vi "LVDatasetTest.vi"() -> ()   [LabVIEW 2011]
uses:
  JelmersTracker.llb/TrackerDLL.vi
  <vilib>/Utility/file.llb/Read From Spreadsheet File (DBL).vi
  <vilib>/Utility/file.llb/Write To Spreadsheet File (DBL).vi
panel:
  out "C++ QI error":cluster{dbl, dbl}(graph)
  out "LV Z":cluster{"Normalized Z":sgl, sgl}(graph)
  out "True pos":dbl(graph)
  out "LV ZLUT":dbl[][](graph)
  out "JTrk ZLUT":sgl[][](graph)
  in  "XCorWindow":u32=64
  out "FPS":dbl
  in  "Use LV tracker":bool=TRUE
  in  "xcor profile":i32=32
  in  "result output dir":string="dataset_result\\roi80"
  out "LV COM error":cluster{dbl, dbl}(graph)
  out "LV QI error":cluster{dbl, dbl}(graph)
  out "LV XCor X&Y error":cluster{dbl, dbl}(graph)
  out "X Resolution":i32
  out "Image Type":T1 items=["Grayscale (U8)", "Grayscale (I16)", "Grayscale (SGL)", "Complex (CSG)", "RGB (U32)", "HSL (U32)", "RGB (U64)", "Grayscale (U16)"]
  in  "LVTracker settings":T2={"Rmax (pix)"=50, "RminZ (pix)"=5, "angular pixel\n coverage factor"=0.7, "radial pixel\n coverage factor"=3.0}
  out "Debug output":sgl[][](graph)
  out "COM X & Y error":cluster{dbl, dbl}(graph)
  out "text file path":path
  out "File":string caption="Result"
  in  "Image count":i32=200
  out "Image":T3(plugin-control)
  in  "xcor_iterations":i32=1
  out "Radial profile":sgl[](graph)
  in  "Path":path=path "D:/jcnossen1/ztracker/Qpaper_007LUT_varyRoi80/tmp_002"
  in  "Browse?":bool=TRUE
  in  "debug library":bool=TRUE
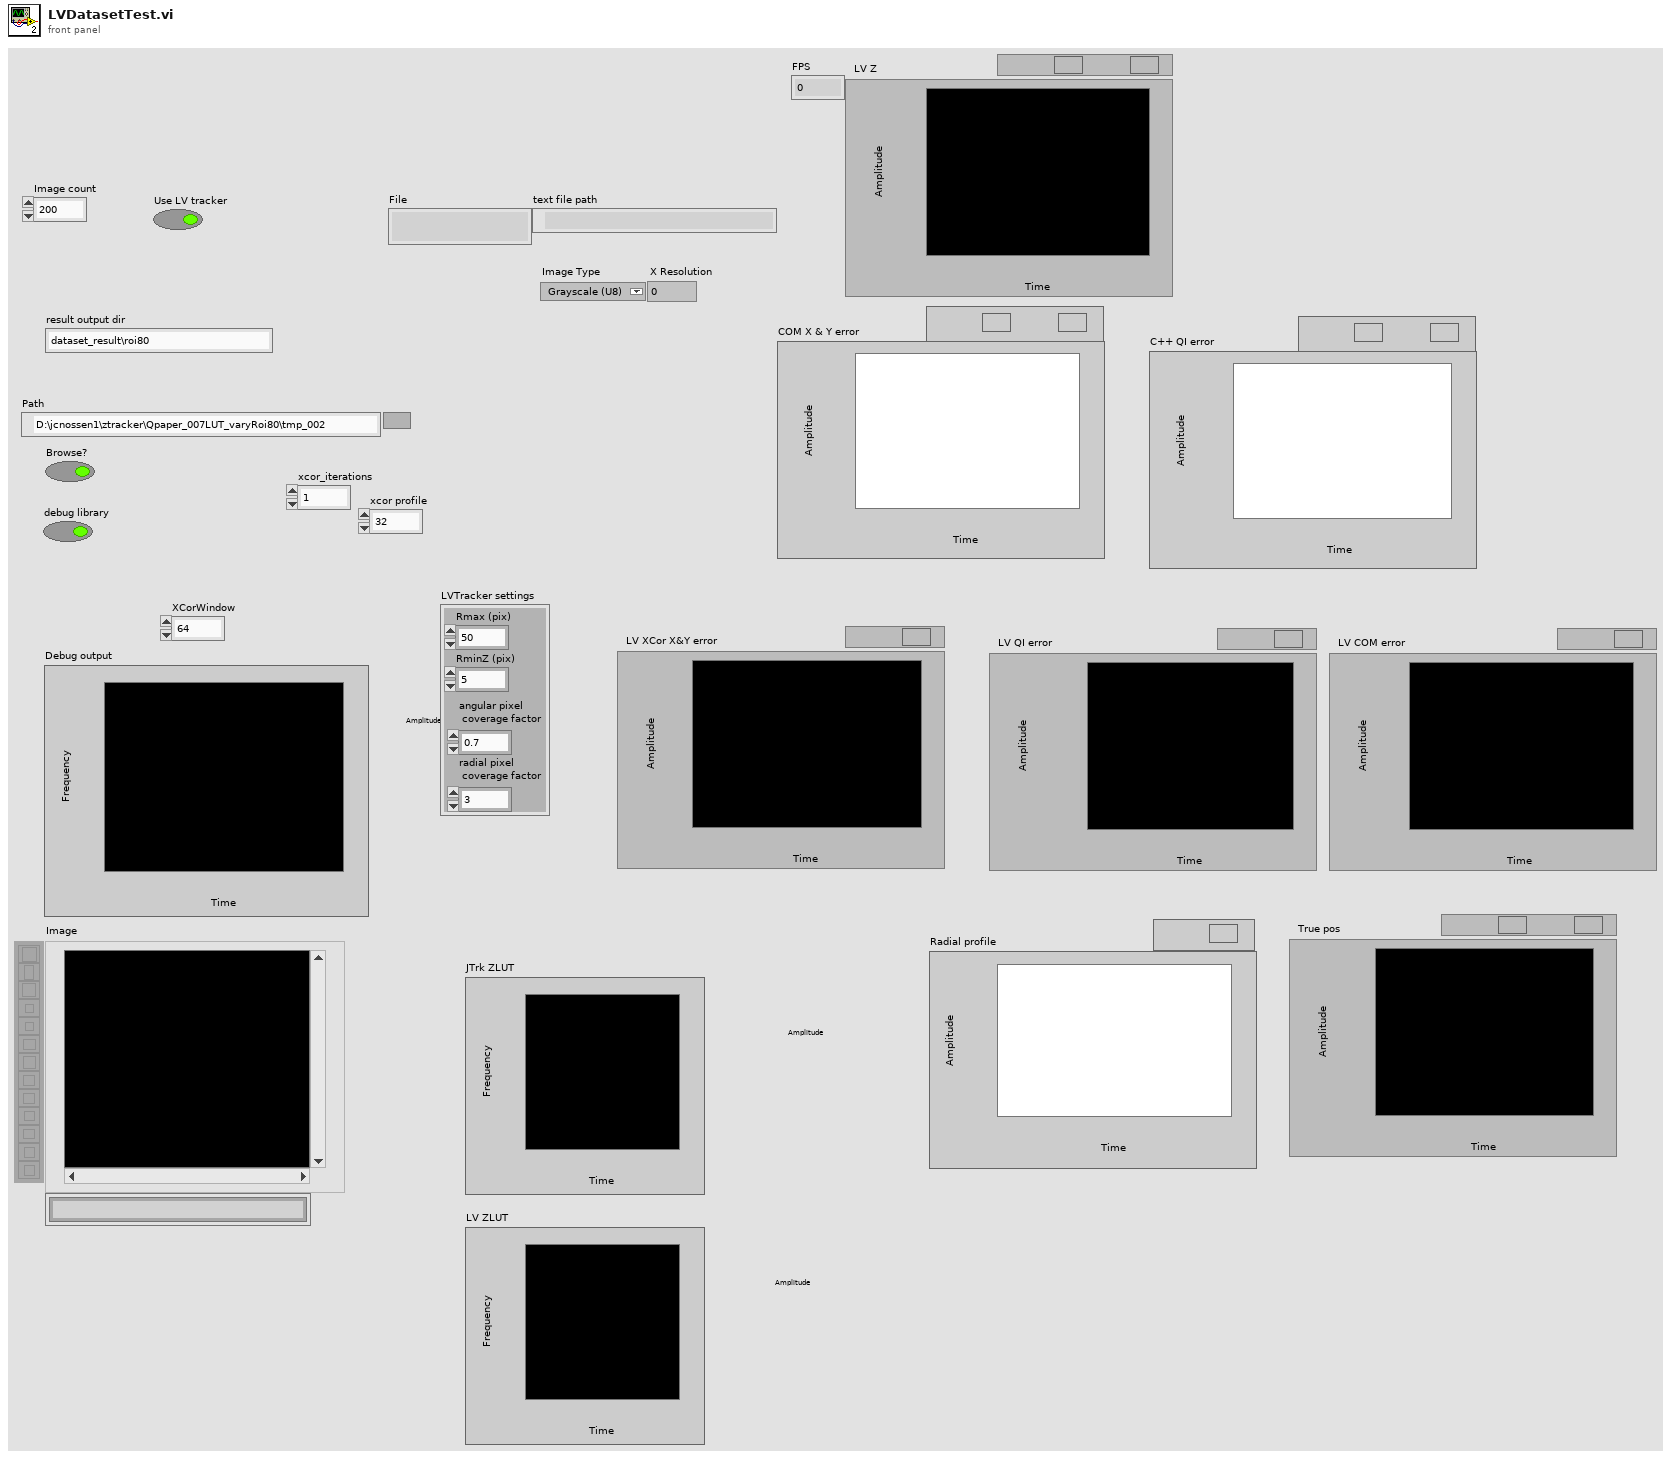
[diagram p1: front panel]
types:
  T1 = typedef "Image Type" = u32
  T2 = cluster{"Rmax (pix)":i32, "RminZ (pix)":i32, "angular pixel\n coverage factor":dbl, "radial pixel\n coverage factor":dbl}
  T3 = typedef "IMAQ Image.ctl" = refnum<image>
  T4 = typedef "TrackerInstance.ctl" = cluster{"Tracker Pointer":u64, "Image size":cluster{"width":u32, "height":u32}}
  T5 = cluster{"New Position (pixels)[0]":dbl, "New Position (pixels)[1]":dbl}
  T6 = cluster{"COM Position (pixels)[0]":dbl, "COM Position (pixels)[1]":dbl}
  T7 = cluster{"XCor coordinates[0]":dbl, "XCor coordinates[1]":dbl}
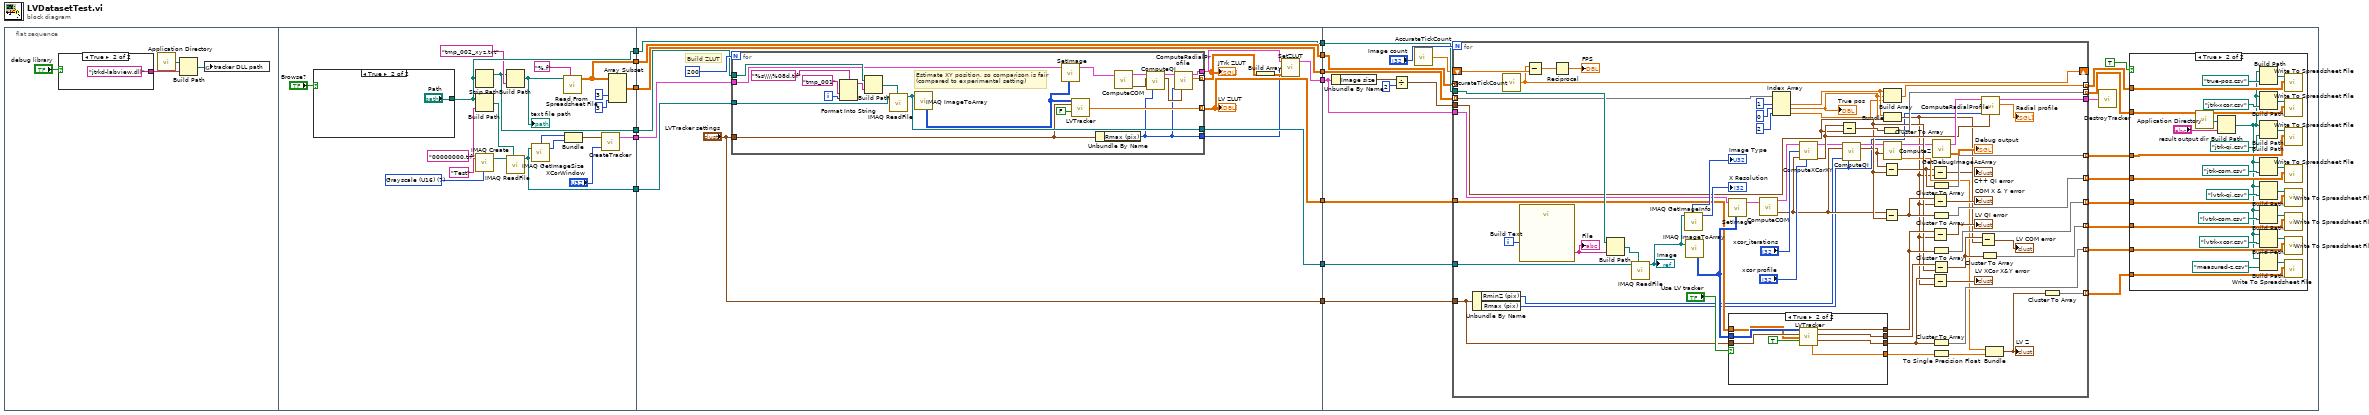
[diagram p0: block diagram]
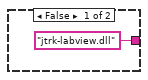
[diagram p2: hidden frame]
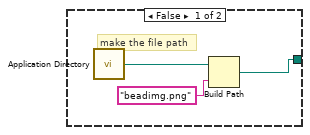
[diagram p3: hidden frame]
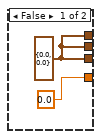
[diagram p5: hidden frame]
diagram:
  n1 = flat-sequence {
    tunnel: [w32] -> w13
    tunnel: [w34] -> w11
    tunnel: [w33] -> w9
    tunnel: [w27] -> w7
    tunnel: [w22] -> w5
    tunnel: [w20] -> w3
    tunnel: w13 -> [w56]
    tunnel: [w56] -> w12
    tunnel: w11 -> [w53]
    tunnel: [w48] -> w10
    tunnel: w9 -> [w54]
    tunnel: [w52] -> w8
    tunnel: w7 -> [w59]
    tunnel: [w59] -> w6
    tunnel: w5 -> [w58]
    tunnel: [w58] -> w4
    tunnel: w3 -> [w55]
    tunnel: ["LVTracker settings"] -> w2
    tunnel: [w50] -> w1
    tunnel: w12 -> [w101]
    tunnel: w10 -> [w92]
    tunnel: w8 -> [w100]
    tunnel: w6 -> [w98]
    tunnel: w4 -> [w94]
    tunnel: w2 -> [w91]
    tunnel: w1 -> [w90]
    frame #0 {
      n2 = case shown="True" "debug library" {
        tunnel: ["jtrk-labview.dll" "jtrkd-labview.dll"] -> w15
        frame False {
        }
        frame True {
        }
      }
      n3 = call <vilib>:"Application Directory.vi"() -> ("Application Directory"=w16:path)
      n4 = Build Path(base path=w16, name or relative path=w15) -> (appended path=w14:path)
      n5 = global write "TrackerDLL.vi" "tracker DLL path"(w14) -> ()
    }
    frame #1 {
      w39 = T1 7 items=["Grayscale (U8)", "Grayscale (I16)", "Grayscale (SGL)", "Complex (CSG)", "RGB (U32)", "HSL (U32)", "RGB (U64)", "Grayscale (U16)"] ("Image Type")
      n6 = case shown="True" "Browse?" {
        tunnel: [w41 "Path"] -> w32
        frame False {
          # "make the file path"
          n7 = call <vilib>:"Application Directory.vi"() -> ("Application Directory"=w42:path)
          n8 = Build Path(base path=w42, name or relative path="beadimg.png") -> (appended path=w41:path)
        }
        frame True {
        }
      }
      n9 = Strip Path(path=w32) -> (stripped path=w20:path)  [unwired: 1 out]
      n10 = Build Path(base path=w32, name or relative path="00000000.tif") -> (appended path=w35:path)
      n11 = call "IMAQ Create"("Image Name"="Test" ("String"), "Image Type"=w39) -> ("New Image"=w36:T3)  [unwired: 3 in, 1 out]
      n12 = Build Path(base path=w20, name or relative path="tmp_002_xyz.txt") -> (appended path=w30:path)
      "text file path" <- w30
      n13 = call "IMAQ ReadFile"("File Path"=w35, "Image"=w36) -> ("Image Out"=w33:T3)  [unwired: 5 in, 4 out]
      n14 = call "IMAQ GetImageSize"("Image"=w33) -> ("Y Resolution"=w24:i32, "X Resolution"=w26:i32)  [unwired: 3 in, 1 out]
      n15 = call-poly <vilib>:"Read From Spreadsheet File.vi"("format (%.3f)"="%.f", "file path (dialog if empty)"=w30) -> ("all rows"=w22:dbl[][])  [unwired: 5 in, 4 out]
      n16 = Bundle("X Resolution"=w26, "Y Resolution"=w24) -> (w25:cluster{"X Resolution":i32, "Y Resolution":i32})  [unwired: 1 in]
      n17 = call "CreateTracker.vi"("XCorWindow"="XCorWindow", "Image size"=w25) -> ("tracker"=w34:T4)  [unwired: 1 in]
      n18 = Array Subset(array=w22, index (col)=3 ("index"), length (col)=3 ("length")) -> (w27:dbl[][])  [unwired: 2 in]
    }
    frame #2 {
      # "Build ZLUT"
      n19 = for {
        N: 200 -> [_]
        tunnel: w55 -> [w80]
        tunnel: w54 -> [w79]
        tunnel: w53 -> [w67]
        tunnel: [w77] -> w52
        tunnel: [w76] -> w49
        tunnel: [w75] -> w47 mode=indexing
        tunnel: "LVTracker settings" -> [w61]
        tunnel: [w62] -> w50 mode=indexing
        tunnel: [w60] -> w45
        i -> [w72]
        # "Estimate XY position, so comparison is fair\n(compared to experimental setting)"
        n20 = Format Into String(format string="%s\\\\%08d.tif", "tmp_001" ("Prefix"), w72) -> (resulting string=w71:string)  [unwired: 2 in, 1 out]
        n21 = Build Path(base path=w80, name or relative path=w71) -> (appended path=w78:path)
        n22 = call "IMAQ ReadFile"("File Path"=w78, "Image"=w79) -> ("Image Out"=w77:T3)  [unwired: 5 in, 4 out]
        n23 = call "IMAQ ImageToArray"("Image"=w77) -> ("Image Pixels (U16)"=w70:u16[][])  [unwired: 3 in, 4 out]
        n24 = call "SetImage.vi"("tracker"=w67, "Image (U16)"=w70) -> ("tracker"=w68:T4)  [unwired: 6 in, 1 out]
        n25 = call "LVTracker.vi"("image in"=w70, "settings"=w61, "Compute Z"=FALSE) -> ("LV tracker rad prof"=w62:dbl[])  [unwired: 7 in, 5 out]
        n26 = Unbundle By Name(w61) -> ("Rmax (pix)"=w60:i32)
        n27 = call "ComputeCOM.vi"("tracker"=w68) -> ("tracker"=w66:T4, "position"=w64:cluster{"X":sgl, "Y":sgl})  [unwired: 2 in]
        n28 = call "ComputeQI.vi"("tracker"=w66, "initial position"=w64, "maxRadius"=w60) -> ("tracker"=w65:T4, "position"=w63:cluster{"X":sgl, "Y":sgl})  [unwired: 10 in, 1 out]
        n29 = call "ComputeRadialProfile.vi"("center"=w63, "radius"=w60, "tracker"=w65) -> ("output"=w75:sgl[], "tracker"=w76:T4)  [unwired: 7 in]
      }
      "JTrk ZLUT" <- w47
      "LV ZLUT" <- w50
      n30 = Build Array(w47) -> (w46:sgl[][][])
      n31 = call "SetZLUT.vi"("zluts"=w46, "profile_radius"=w45, "tracker instance"=w49) -> ("tracker"=w48:T4)  [unwired: 2 in]
    }
    frame #3 {
      n32 = Unbundle By Name(w92) -> ("Image size"=w97:cluster{"width":u32, "height":u32})
      n33 = Divide(x=w97, y=2) -> (x/y=w95:cluster{"width":dbl, "height":dbl})
      n34 = call "AccurateTickCount.vi"() -> ("seconds"=w93:dbl)
      n35 = for {
        N: "Image count" -> [_]
        tunnel: w101 -> [w193]
        tunnel: w92 -> [w157]
        tunnel: w100 -> [w190]
        tunnel: [w181] -> w99
        tunnel: w98 -> [w189] mode=indexing
        tunnel: w95 -> [w153]
        tunnel: [w180] -> w84 mode=indexing
        tunnel: [w178] -> w87 mode=indexing
        tunnel: [w173] -> w89 mode=indexing
        tunnel: [w171] -> w83 mode=indexing
        tunnel: [w169] -> w88 mode=indexing
        tunnel: w94 -> [_] mode=indexing
        shift-right: [w159] -> _
        shift-left: w93 -> [w162]
        tunnel: [w152] -> w86 mode=indexing
        tunnel: w91 -> [w135]
        tunnel: w90 -> [w149]
        tunnel: [w140] -> w85 mode=indexing
        tunnel: [w138] -> w82 mode=indexing
        i -> [w191]
        n36 = Unbundle By Name(w135) -> ("RminZ (pix)"=w134:i32, "Rmax (pix)"=w130:i32)
        n37 = call "AccurateTickCount.vi"() -> ("seconds"=w159:dbl)
        n38 = call "Build Text"("ImageNumber"=w191) -> ("Result"=w194:string)  [unwired: 13 in, 1 out]
        "File" <- w194
        n39 = Subtract(x=w159, y=w162) -> (x-y=w161:dbl)
        n40 = Reciprocal(x=w161) -> (1/x=→"FPS":dbl)
        n41 = Build Path(base path=w193, name or relative path=w194) -> (appended path=w192:path)
        n42 = call "IMAQ ReadFile"("File Path"=w192, "Image"=w190) -> ("Image Out"=w158:T3)  [unwired: 5 in, 4 out]
        "Image" <- w158
        n43 = call "IMAQ GetImageInfo"("Image"=w158) -> ("X Resolution"=→"X Resolution":i32, "Image Type"=→"Image Type":T1)  [unwired: 3 in, 6 out]
        n44 = call "IMAQ ImageToArray"("Image"=w158) -> ("Image Pixels (U16)"=w155:u16[][])  [unwired: 3 in, 4 out]
        n45 = call "SetImage.vi"("tracker"=w157, "Image (U16)"=w155) -> ("tracker"=w156:T4)  [unwired: 6 in, 1 out]
        n46 = case shown="True" "Use LV tracker" {
          tunnel: w135 -> [_ w205]
          tunnel: [w197 w203] -> w175
          tunnel: [w197 w201] -> w168
          tunnel: [w197 w202] -> w150
          tunnel: w155 -> [_ w204]
          tunnel: w149 -> [_ w200]
          tunnel: [0.0 ("New Position (pixels)[1]") w198] -> w136
          frame False {
            w197 = T5 {"New Position (pixels)[0]"=0.0, "New Position (pixels)[1]"=0.0} ("qi position")
          }
          frame True {
            n47 = call "LVTracker.vi"("image in"=w204, "settings"=w205, "Z LUT"=w200, "Compute Z"=TRUE) -> ("qi position"=w201:T5, "com position"=w203:T6, "xcor position"=w202:T7, "Z plane index"=w198:dbl)  [unwired: 6 in, 2 out]
          }
        }
        n48 = call "ComputeCOM.vi"("tracker"=w156) -> ("tracker"=w186:T4, "position"=w151:cluster{"X":sgl, "Y":sgl})  [unwired: 2 in]
        n49 = Index Array(array=w189, index #1=1 ("index"), index #2=0 ("index"), index #3=2 ("index")) -> (element #1=w143:dbl, element #2=w142:dbl, element #3=w141:dbl)
        "True pos" <- w142
        n50 = call "ComputeXCorXY.vi"("tracker"=w186, "iterations"="xcor_iterations", "position"=w151, "profileWidth"="xcor profile") -> ("tracker"=w154:T4, "position"=w182:cluster{"X":sgl, "Y":sgl})  [unwired: 1 in, 2 out]
        n51 = Subtract(x=w182, y=w153) -> (x-y=w166:cluster{dbl, dbl})
        n52 = call "ComputeQI.vi"("tracker"=w154, "initial position"=w151, "minRadius"=w134, "maxRadius"=w130) -> ("tracker"=w147:T4, "position"=w146:cluster{"X":sgl, "Y":sgl})  [unwired: 9 in, 1 out]
        n53 = Cluster To Array(cluster=w166) -> (array=w180:dbl[])
        n54 = Subtract(x=w146, y=w153) -> (x-y=w133:cluster{dbl, dbl})
        n55 = Subtract(x=w151, y=w153) -> (x-y=w165:cluster{dbl, dbl})
        n56 = Build Array(w143, w142, w141) -> (w140:dbl[])
        n57 = Bundle(w143, w142) -> (w132:cluster{dbl, dbl})  [unwired: 1 in]
        n58 = call "ComputeZ.vi"("position"=w146, "tracker instance"=w147) -> ("Normalized Z"=w145:sgl, "tracker instance"=w148:T4)  [unwired: 4 in]
        n59 = Subtract(x=w133, y=w132) -> (x-y=→"C++ QI error":cluster{dbl, dbl})
        n60 = Subtract(x=w165, y=w132) -> (x-y=→"COM X & Y error":cluster{dbl, dbl})
        n61 = Subtract(x=w168, y=w132) -> (x-y=→"LV QI error":cluster{dbl, dbl})
        n62 = Subtract(x=w150, y=w132) -> (x-y=→"LV XCor X&Y error":cluster{dbl, dbl})
        n63 = Cluster To Array(cluster=w133) -> (array=w152:dbl[])
        n64 = Cluster To Array(cluster=w165) -> (array=w178:dbl[])
        n65 = Cluster To Array(cluster=w168) -> (array=w171:dbl[])
        n66 = Subtract(x=w175, y=w153) -> (x-y=w167:cluster{dbl, dbl})
        n67 = Cluster To Array(cluster=w150) -> (array=w173:dbl[])
        n68 = call "GetDebugImageAsArray.vi"("tracker"=w148) -> ("image"=→"Debug output":sgl[][], "tracker"=w185:T4)  [unwired: 1 in]
        n69 = To Single Precision Float(number=w136) -> (single precision float=w137:sgl)
        n70 = Subtract(x=w167, y=w132) -> (x-y=→"LV COM error":cluster{dbl, dbl})
        n71 = Cluster To Array(cluster=w167) -> (array=w169:dbl[])
        n72 = call "ComputeRadialProfile.vi"("center"=w182, "radius"=w130, "tracker"=w185) -> ("output"=→"Radial profile":sgl[], "tracker"=w181:T4)  [unwired: 7 in]
        n73 = Bundle("Normalized Z"=w145, w137) -> (w139:cluster{"Normalized Z":sgl, sgl})  [unwired: 1 in]
        "LV Z" <- w139
        n74 = Cluster To Array(cluster=w139) -> (array=w138:sgl[])
      }
      n75 = call "DestroyTracker.vi"("tracker instance"=w99) -> ()
      n76 = case shown="True" TRUE {
        tunnel: w89 -> [_ w113]
        tunnel: w88 -> [_ w112]
        tunnel: w87 -> [_ w111]
        tunnel: w86 -> [_ w110]
        tunnel: w85 -> [_ w109]
        tunnel: w84 -> [_ w108]
        tunnel: w83 -> [_ w107]
        tunnel: w82 -> [_ w104]
        frame False {
        }
        frame True {
          n77 = call <vilib>:"Application Directory.vi"() -> ("Application Directory"=w126:path)
          n78 = Build Path(base path=w126, name or relative path="result output dir") -> (appended path=w105:path)
          n79 = Build Path(base path=w105, name or relative path=path "true-pos.csv" ("file path (dialog if empty)")) -> (appended path=w125:path)
          n80 = Build Path(base path=w105, name or relative path=path "jtrk-xcor.csv" ("file path (dialog if empty)")) -> (appended path=w116:path)
          n81 = Build Path(base path=w105, name or relative path=path "jtrk-qi.csv" ("file path (dialog if empty)")) -> (appended path=w129:path)
          n82 = Build Path(base path=w105, name or relative path=path "jtrk-com.csv" ("file path (dialog if empty)")) -> (appended path=w122:path)
          n83 = Build Path(base path=w105, name or relative path=path "lvtrk-qi.csv" ("file path (dialog if empty)")) -> (appended path=w120:path)
          n84 = Build Path(base path=w105, name or relative path=path "lvtrk-com.csv" ("file path (dialog if empty)")) -> (appended path=w123:path)
          n85 = Build Path(base path=w105, name or relative path=path "lvtrk-xcor.csv" ("file path (dialog if empty)")) -> (appended path=w114:path)
          n86 = Build Path(base path=w105, name or relative path=path "measured-z.csv" ("file path (dialog if empty)")) -> (appended path=w103:path)
          n87 = call-poly <vilib>:"Write To Spreadsheet File.vi"("2D data"=w109, "file path (dialog if empty)"=w125) -> ()  [unwired: 6 in, 1 out]
          n88 = call-poly <vilib>:"Write To Spreadsheet File.vi"("2D data"=w108, "file path (dialog if empty)"=w116) -> ()  [unwired: 6 in, 1 out]
          n89 = call-poly <vilib>:"Write To Spreadsheet File.vi"("2D data"=w110, "file path (dialog if empty)"=w129) -> ()  [unwired: 6 in, 1 out]
          n90 = call-poly <vilib>:"Write To Spreadsheet File.vi"("2D data"=w111, "file path (dialog if empty)"=w122) -> ()  [unwired: 6 in, 1 out]
          n91 = call-poly <vilib>:"Write To Spreadsheet File.vi"("2D data"=w107, "file path (dialog if empty)"=w120) -> ()  [unwired: 6 in, 1 out]
          n92 = call-poly <vilib>:"Write To Spreadsheet File.vi"("2D data"=w112, "file path (dialog if empty)"=w123) -> ()  [unwired: 6 in, 1 out]
          n93 = call-poly <vilib>:"Write To Spreadsheet File.vi"("2D data"=w113, "file path (dialog if empty)"=w114) -> ()  [unwired: 6 in, 1 out]
          n94 = call-poly <vilib>:"Write To Spreadsheet File.vi"("2D data"=w104, "file path (dialog if empty)"=w103) -> ()  [unwired: 6 in, 1 out]
        }
      }
    }
  }
